vi "dfd_Build Waveform Graph.vi"(5 "fs":dbl=1.0, 7 "# freq bins out":i32, 10 "values":dbl[](array[numeric]), 11 "f0":dbl) -> (3 "waveform":cluster{"f0":dbl, "df":dbl, "values":dbl[]})   [LabVIEW 2017, in "NI_DigFilter_FilterBank.lvlib"]
uses:
  <vilib>/addons/Digital Filter Design/NI_DigFilter_FilterBank.lvlib
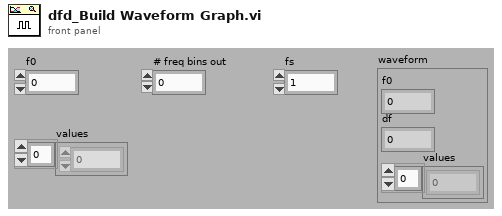
[diagram p1: front panel]
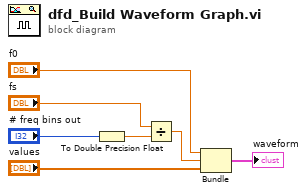
[diagram p0: block diagram]
diagram:
  n1 = To Double Precision Float(number="# freq bins out") -> (double precision float=w2:dbl)
  n2 = Divide(x="fs", y=w2) -> (x/y=w1:dbl)
  n3 = Bundle("f0"="f0", w1, "values"="values") -> (→"waveform":cluster{"f0":dbl, dbl, "values":dbl[]})  [unwired: 1 in]
